vi "S2C_PCIe7841_Proc_DigitalRead.vi"(8 "Error In":errorcluster, 11 "Data":string) -> (0 "Error Out":errorcluster, 3 "Response":string)   [LabVIEW 2015]
uses:
  Typedefs/S2C_PCIe7841_Type_Conn0.ctl
  Typedefs/S2C_PCIe7841_Type_Conn1.ctl
  Typedefs/S2C_PCIe7841_Type_Conn2.ctl
  S2C_PCIe7841_Proc_Globals.vi
  <vilib>/Utility/error.llb/Error Cluster From Error Code.vi
  <vilib>/rvi/errors/niLvFpgaAdjustHostInterfaceError.vi
  <vilib>/rvi/interface/nirviReadWriteControl/nirviReadWriteControl.xnode
  NiFpgaLv.dll
  <vilib>/rvi/interface/Simulation/niFpgaSimulationCallBeginRW.vi
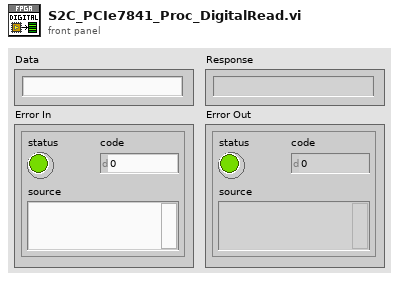
[diagram p1: front panel]
types:
  T1 = typedef "S2C_PCIe7841_Type_Conn0.ctl" = u16
  T2 = typedef "S2C_PCIe7841_Type_Conn1.ctl" = u16
  T3 = typedef "S2C_PCIe7841_Type_Conn2.ctl" = u16
  T4 = cluster{"Connector":u16, "Conn0_Item":T1, "Conn1_Item":T2, "Conn2_Item":T3}
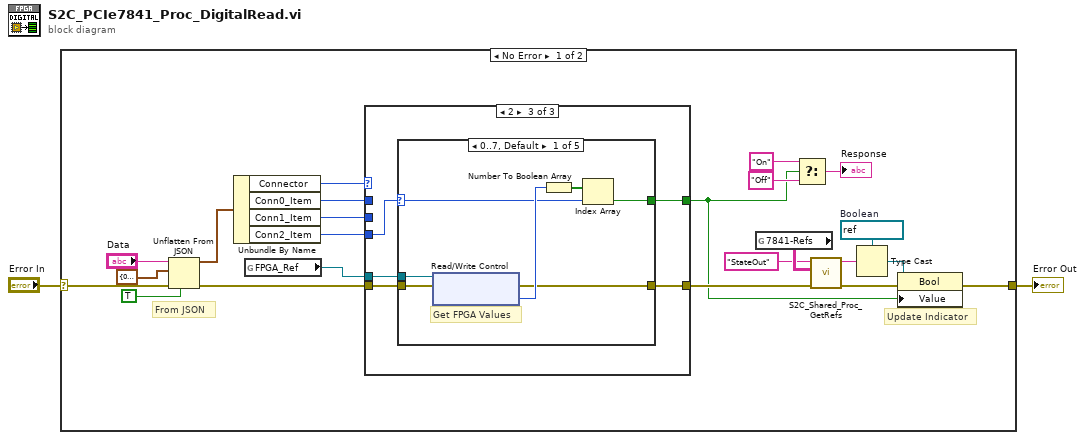
[diagram p0: block diagram]
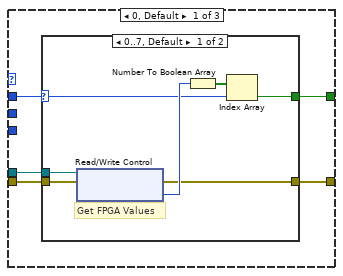
[diagram p2: hidden frame]
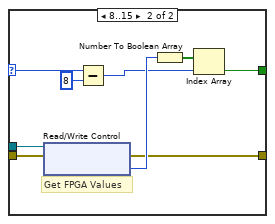
[diagram p3: hidden frame]
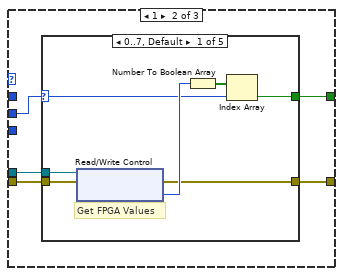
[diagram p4: hidden frame]
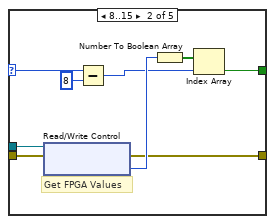
[diagram p5: hidden frame]
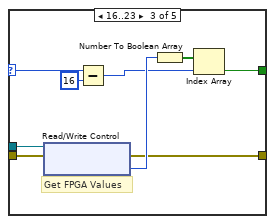
[diagram p6: hidden frame]
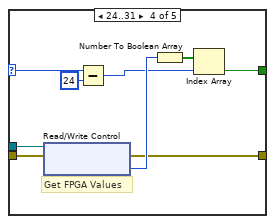
[diagram p7: hidden frame]
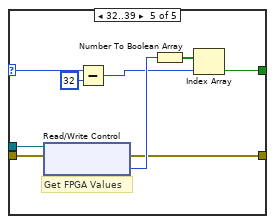
[diagram p8: hidden frame]
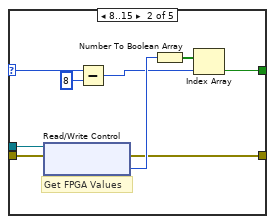
[diagram p9: hidden frame]
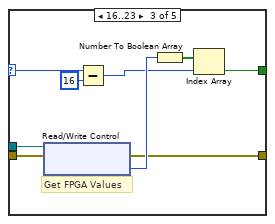
[diagram p10: hidden frame]
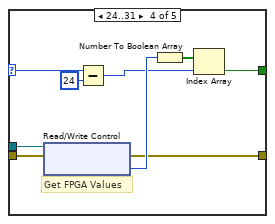
[diagram p11: hidden frame]
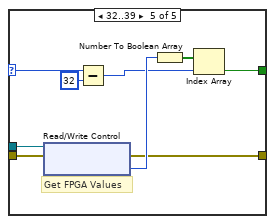
[diagram p12: hidden frame]
diagram:
  n1 = case shown="No Error" "Error In" {
    selector: "Error In" -> [w25 w143]
    tunnel: [w4 w143] -> w1
    frame No Error {
      w10 = refnum<vi> refnum  # Boolean
      # "Update Indicator"
      # "From JSON"
      n2 = Unflatten From JSON(JSON string="Data", type and defaults=T4 {"Connector"=0, "Conn0_Item"=14, "Conn1_Item"=0, "Conn2_Item"=0}, default null elements? (F)=TRUE, error in (no error)=w25) -> (value=w22:T4, error out=w19:errorcluster)  [unwired: 3 in]
      n3 = Unbundle By Name(w22) -> ("Connector"=w21:u16, "Conn0_Item"=w18:T1, "Conn1_Item"=w17:T2, "Conn2_Item"=w16:T3)
      n4 = global read "S2C_PCIe7841_Proc_Globals.vi" "FPGA_Ref"() -> (w15:refnum<k20>)
      n5 = case shown="2" w21 {
        tunnel: w19 -> [w30 w51 w99]
        tunnel: w18 -> [w29 _ _]
        tunnel: w17 -> [_ w47 _]
        tunnel: w16 -> [_ _ w95]
        tunnel: w15 -> [w28 w50 w98]
        tunnel: [w27 w49 w97] -> w6
        tunnel: [w26 w48 w96] -> w9
        frame 0, Default {
          n6 = case shown="0..7, Default" w29 {
            selector: w29 -> [w33 w41]
            tunnel: w30 -> [w37 w46]
            tunnel: w28 -> [w36 w45]
            tunnel: [w32 w42] -> w27
            tunnel: [w31 w38] -> w26
            frame 0..7, Default {
              # "Get FPGA Values"
              n7 = xnode "Read/Write Control"("FPGA VI Reference In"=w36, "error in"=w37) -> ("error out"=w31:errorcluster, "Conn0/Port0"=w35:u8)  [unwired: 1 out]
              n8 = Number To Boolean Array(number=w35) -> (Boolean array=w34:bool[])
              n9 = Index Array(array=w34, index=w33) -> (element=w32:bool)
            }
            frame 8..15 {
              # "Get FPGA Values"
              n10 = xnode "Read/Write Control"("FPGA VI Reference In"=w45, "error in"=w46) -> ("error out"=w38:errorcluster, "Conn0/Port1"=w44:u8)  [unwired: 1 out]
              n11 = Subtract(x=w41, y=8) -> (x-y=w39:i32)
              n12 = Number To Boolean Array(number=w44) -> (Boolean array=w43:bool[])
              n13 = Index Array(array=w43, index=w39) -> (element=w42:bool)
            }
          }
        }
        frame 1 {
          n14 = case shown="0..7, Default" w47 {
            selector: w47 -> [w54 w62 w71 w80 w89]
            tunnel: w51 -> [w58 w67 w76 w85 w94]
            tunnel: w50 -> [w57 w66 w75 w84 w93]
            tunnel: [w53 w63 w72 w81 w90] -> w49
            tunnel: [w52 w59 w68 w77 w86] -> w48
            frame 0..7, Default {
              # "Get FPGA Values"
              n15 = xnode "Read/Write Control"("FPGA VI Reference In"=w57, "error in"=w58) -> ("error out"=w52:errorcluster, "Conn1/Port0"=w56:u8)  [unwired: 1 out]
              n16 = Number To Boolean Array(number=w56) -> (Boolean array=w55:bool[])
              n17 = Index Array(array=w55, index=w54) -> (element=w53:bool)
            }
            frame 8..15 {
              # "Get FPGA Values"
              n18 = xnode "Read/Write Control"("FPGA VI Reference In"=w66, "error in"=w67) -> ("error out"=w59:errorcluster, "Conn1/Port1"=w65:u8)  [unwired: 1 out]
              n19 = Subtract(x=w62, y=8) -> (x-y=w60:i32)
              n20 = Number To Boolean Array(number=w65) -> (Boolean array=w64:bool[])
              n21 = Index Array(array=w64, index=w60) -> (element=w63:bool)
            }
            frame 16..23 {
              # "Get FPGA Values"
              n22 = xnode "Read/Write Control"("FPGA VI Reference In"=w75, "error in"=w76) -> ("error out"=w68:errorcluster, "Conn1/Port2"=w74:u8)  [unwired: 1 out]
              n23 = Subtract(x=w71, y=16) -> (x-y=w69:i32)
              n24 = Number To Boolean Array(number=w74) -> (Boolean array=w73:bool[])
              n25 = Index Array(array=w73, index=w69) -> (element=w72:bool)
            }
            frame 24..31 {
              # "Get FPGA Values"
              n26 = xnode "Read/Write Control"("FPGA VI Reference In"=w84, "error in"=w85) -> ("error out"=w77:errorcluster, "Conn1/Port3"=w83:u8)  [unwired: 1 out]
              n27 = Subtract(x=w80, y=24) -> (x-y=w78:i32)
              n28 = Number To Boolean Array(number=w83) -> (Boolean array=w82:bool[])
              n29 = Index Array(array=w82, index=w78) -> (element=w81:bool)
            }
            frame 32..39 {
              # "Get FPGA Values"
              n30 = xnode "Read/Write Control"("FPGA VI Reference In"=w93, "error in"=w94) -> ("error out"=w86:errorcluster, "Conn1/Port4"=w92:u8)  [unwired: 1 out]
              n31 = Subtract(x=w89, y=32) -> (x-y=w87:i32)
              n32 = Number To Boolean Array(number=w92) -> (Boolean array=w91:bool[])
              n33 = Index Array(array=w91, index=w87) -> (element=w90:bool)
            }
          }
        }
        frame 2 {
          n34 = case shown="0..7, Default" w95 {
            selector: w95 -> [w102 w110 w119 w128 w137]
            tunnel: w99 -> [w106 w115 w124 w133 w142]
            tunnel: w98 -> [w105 w114 w123 w132 w141]
            tunnel: [w101 w111 w120 w129 w138] -> w97
            tunnel: [w100 w107 w116 w125 w134] -> w96
            frame 0..7, Default {
              # "Get FPGA Values"
              n35 = xnode "Read/Write Control"("FPGA VI Reference In"=w105, "error in"=w106) -> ("error out"=w100:errorcluster, "Conn2/Port0"=w104:u8)  [unwired: 1 out]
              n36 = Number To Boolean Array(number=w104) -> (Boolean array=w103:bool[])
              n37 = Index Array(array=w103, index=w102) -> (element=w101:bool)
            }
            frame 8..15 {
              # "Get FPGA Values"
              n38 = xnode "Read/Write Control"("FPGA VI Reference In"=w114, "error in"=w115) -> ("error out"=w107:errorcluster, "Conn2/Port1"=w113:u8)  [unwired: 1 out]
              n39 = Subtract(x=w110, y=8) -> (x-y=w108:i32)
              n40 = Number To Boolean Array(number=w113) -> (Boolean array=w112:bool[])
              n41 = Index Array(array=w112, index=w108) -> (element=w111:bool)
            }
            frame 16..23 {
              # "Get FPGA Values"
              n42 = xnode "Read/Write Control"("FPGA VI Reference In"=w123, "error in"=w124) -> ("error out"=w116:errorcluster, "Conn2/Port2"=w122:u8)  [unwired: 1 out]
              n43 = Subtract(x=w119, y=16) -> (x-y=w117:i32)
              n44 = Number To Boolean Array(number=w122) -> (Boolean array=w121:bool[])
              n45 = Index Array(array=w121, index=w117) -> (element=w120:bool)
            }
            frame 24..31 {
              # "Get FPGA Values"
              n46 = xnode "Read/Write Control"("FPGA VI Reference In"=w132, "error in"=w133) -> ("error out"=w125:errorcluster, "Conn2/Port3"=w131:u8)  [unwired: 1 out]
              n47 = Subtract(x=w128, y=24) -> (x-y=w126:i32)
              n48 = Number To Boolean Array(number=w131) -> (Boolean array=w130:bool[])
              n49 = Index Array(array=w130, index=w126) -> (element=w129:bool)
            }
            frame 32..39 {
              # "Get FPGA Values"
              n50 = xnode "Read/Write Control"("FPGA VI Reference In"=w141, "error in"=w142) -> ("error out"=w134:errorcluster, "Conn2/Port4"=w140:u8)  [unwired: 1 out]
              n51 = Subtract(x=w137, y=32) -> (x-y=w135:i32)
              n52 = Number To Boolean Array(number=w140) -> (Boolean array=w139:bool[])
              n53 = Index Array(array=w139, index=w135) -> (element=w138:bool)
            }
          }
        }
      }
      n54 = global read "S2C_PCIe7841_Proc_Globals.vi" "7841-Refs"() -> (w14:string[][])
      n55 = Select(t="On" ("Label"), s=w6, f="Off" ("Label")) -> (s? t:f=→"Response":string)
      n56 = call "S2C_Shared_Proc_GetRefs.vi"("Error In"=w9, "Refs"=w14, "Label"="StateOut") -> ("Error Out"=w12:errorcluster, "Reference"=w11:string)  [unwired: 7 in]
      n57 = Type Cast(type=w10, x=w11) -> (*(type *) &x=w13:refnum<vi>)
      n58 = property class="Bool"(reference=w13, error in=w12, "Value"=w6) -> (error out=w4:errorcluster)  [unwired: 1 out]
    }
    frame Error {
    }
  }
  "Error Out" <- w1
